vi "Create Object.vi"(8 "error in (no error)":errorcluster, 10 "Object Attributes":T1, 11 "GObject in":refnum<class "Object.lvclass">) -> (0 "error out":errorcluster, 3 "GObject out":refnum<class "Object.lvclass">)   [LabVIEW 2017, in "Front Panel Publisher.lvlib" / "Object.lvclass"]
uses:
  Object.lvclass
  Web Front Panel_class/Web Front Panel.lvclass
  Coordinates.ctl
  Attributes.ctl
  <vilib>/Utility/miscctls.llb/LVRectTypeDef.ctl
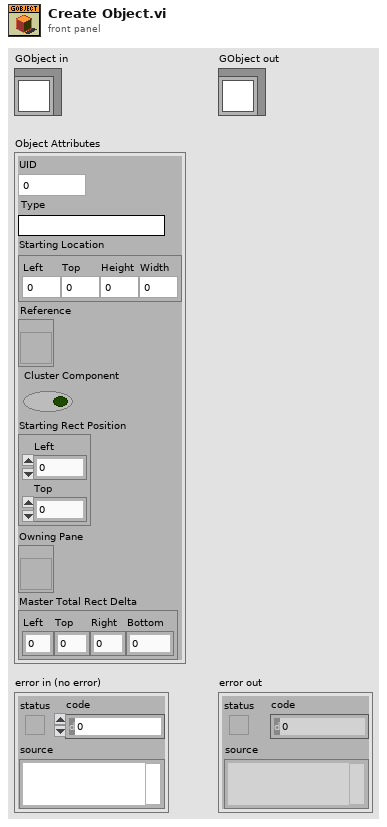
[diagram p1: front panel]
types:
  T1 = typedef "Front Panel Publisher.lvlib/Object.lvclass/Attributes.ctl" = cluster{"UID":i32, "Type":string, "Starting Location":T2, "Reference":refnum<vi>, "Cluster Component":bool, "Starting Rect Position":cluster{"Left":i16, "Top":i16}, "Owning Pane":refnum<vi>, "Master Total Rect Delta":T3}
  T2 = typedef "Front Panel Publisher.lvlib/Object.lvclass/Coordinates.ctl" = cluster{"Left":i32, "Top":i32, "Height":u32, "Width":u32}
  T3 = typedef "LVRectTypeDef.ctl" = cluster{"Left":i16, "Top":i16, "Right":i16, "Bottom":i16}
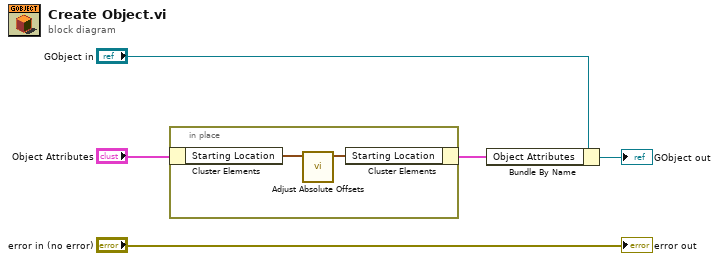
[diagram p0: block diagram]
diagram:
  n1 = in-place {
    n2 = in-place-cluster #1("Object Attributes") -> ("Starting Location"=w7:T2)
    n3 = call "Adjust Absolute Offsets.vi"("Coordinates in"=w7) -> ("Coordinates out"=w6:T2)  [unwired: 8 in, 2 out]
    n4 = in-place-cluster #1("Starting Location"=w6) -> (w1:T1)
  }
  n5 = Bundle By Name(cluster="GObject in", "Object Attributes"=w1) -> (→"GObject out":refnum<class "Object.lvclass">)
  "error out" <- "error in (no error)"
